vi "angleconv.vi"(10 "deg":dbl, 11 "rad":dbl) -> (2 "rad":dbl, 3 "deg":dbl)   [LabVIEW 2015]
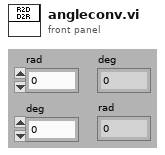
[diagram p1: front panel]
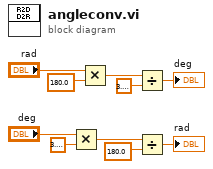
[diagram p0: block diagram]
diagram:
  n1 = Multiply(x="deg", y=3.141592653589793) -> (x*y=w5:dbl)
  n2 = Multiply(x="rad", y=180.0) -> (x*y=w8:dbl)
  n3 = Divide(x=w8, y=3.141592653589793) -> (x/y=→"deg":dbl)
  n4 = Divide(x=w5, y=180.0) -> (x/y=→"rad":dbl)
